vi "数据表-获取全部.vi"(7 "元素名[]-累积记录":string[](array[string]), 8 "error in (no error)":errorcluster, 10 "table":string, 11 "数据库引用":T2) -> (0 "error out":errorcluster, 2 "累积记录数据":T1[](array[typedef]), 3 "connection reference out":T2)   [LabVIEW 2017]
uses:
  <vilib>/addons/database/Connection.llb/Conn ObjectReference.ctl
  <vilib>/addons/database/_DB Variant To Data/Database Variant To Data.xnode
  <vilib>/addons/database/NI_Database_API.lvlib
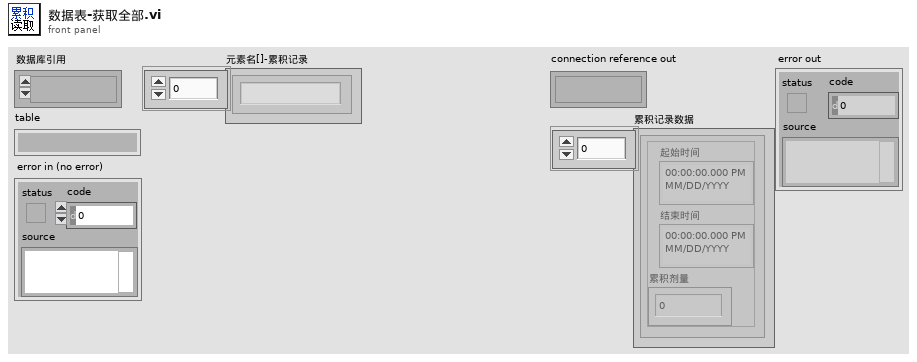
[diagram p1: front panel]
types:
  T1 = typedef "单条累积记录.ctl" = cluster{"起始时间":timestamp, "结束时间":timestamp, "累积剂量":dbl}
  T2 = typedef "NI_Database_API.lvlib/Conn ObjectReference.ctl" = refnum<k1>
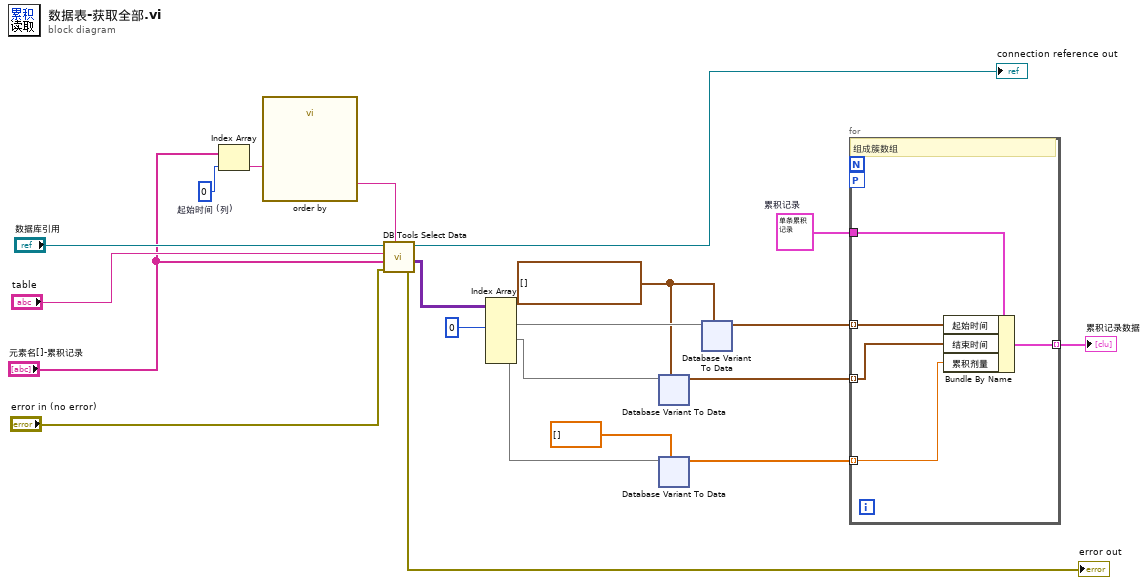
[diagram p0: block diagram]
diagram:
  w3 = 0  # 起始时间 (列)
  w10 = T1 {"起始时间"=timestamp(0 s since 1904-01-01), "结束时间"=timestamp(0 s since 1904-01-01), "累积剂量"=0.0}  # 累积记录
  w12 = timestamp[] []
  n1 = Index Array(array="元素名[]-累积记录", index=w3) -> (element=w4:string)
  n2 = call "order by"("排序列"=w4) -> ("Result"=w2:string)  [unwired: 13 in, 1 out]
  n3 = call <vilib>:"DB Tools Select Data.vi"("condition"=w2, "error in (no error)"="error in (no error)", "columns"="元素名[]-累积记录", "table"="table", "connection reference"="数据库引用") -> ("error out"=→"error out":errorcluster, "data"=w17:variant[][], "connection reference out"=→"connection reference out":T2)  [unwired: 1 in]
  n4 = Index Array(array=w17, index (col) #1=0 ("禁用的索引 (列)")) -> (element #1=w15:variant[], element #2=w14:variant[], element #3=w13:variant[])  [unwired: 5 in]
  n5 = xnode "Database Variant To Data"("database variant"=w14, "type"=w12) -> ("data"=w8:timestamp[])  [unwired: 1 in, 1 out]
  n6 = xnode "Database Variant To Data"("database variant"=w13, "type"=dbl[] []) -> ("data"=w7:dbl[])  [unwired: 1 in, 1 out]
  n7 = xnode "Database Variant To Data"("database variant"=w15, "type"=w12) -> ("data"=w9:timestamp[])  [unwired: 1 in, 1 out]
  n8 = for {
    tunnel: w9 -> [w25] mode=indexing
    tunnel: w8 -> [w24] mode=indexing
    tunnel: w7 -> [w23] mode=indexing
    tunnel: w10 -> [w26]
    tunnel: [w22] -> w6 mode=indexing
    workers-P: _ -> [_]
    # "组成簇数组"
    n9 = Bundle By Name(cluster=w26, "起始时间"=w25, "结束时间"=w24, "累积剂量"=w23) -> (w22:T1)
  }
  "累积记录数据" <- w6
